vi "Create Temporary Location to Store Downloaded Measurement Plugins.vi"(8 "error in (no error)":errorcluster) -> (0 "error out":errorcluster, 3 "created path":path)   [LabVIEW 2013, in "Client Controller.lvlib" / "Client Controller.lvclass"]
uses:
  Client Controller.lvclass
  <vilib>/Utility/sysdir.llb/System Directory Type.ctl
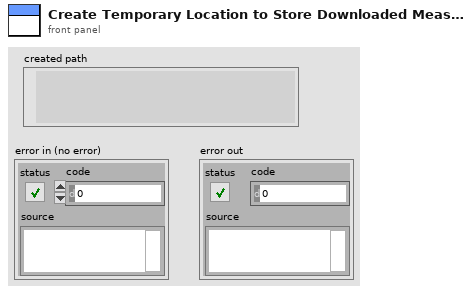
[diagram p1: front panel]
types:
  T1 = typedef "System Directory Type.ctl" = i32
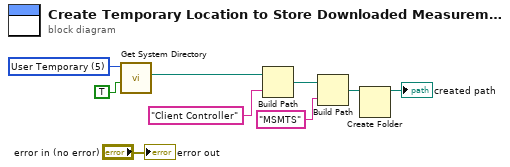
[diagram p0: block diagram]
diagram:
  w3 = T1 5 items=["User Home"=0, "User Desktop"=1, "User Documents"=2, "User Application Data"=3, "User Preferences"=4, "User Temporary"=5, "Public Documents"=6, "Public Application Data"=7, "Public Preferences"=8, "Public Cache"=13, "System Core Libraries"=9, "System Installed Libraries"=10, "Application Files"=11, "Boot Volume Root"=12] ("system directory type")
  n1 = call <vilib>:"Get System Directory.vi"("create directory if not found? (F)"=TRUE, "system directory type"=w3) -> ("system directory"=w5:path)  [unwired: 9 in]
  n2 = Build Path(base path=w5, name or relative path="Client Controller") -> (appended path=w7:path)
  n3 = Build Path(base path=w7, name or relative path="MSMTS") -> (appended path=w9:path)
  n4 = Create Folder(path (use dialog)=w9) -> (created path=→"created path":path)  [unwired: 2 in, 2 out]
  "error out" <- "error in (no error)"
